vi "handle.vi"(5 "TCP connection":refnum<k5>, 7 "response queue":refnum<queue>, 10 "application request in":T1, 11 "http responder in":refnum<class "http responder.lvclass">) -> (0 "stop processing":bool, 3 "http responder out":refnum<class "http responder.lvclass">)   [LabVIEW 2013, in "http responder.lvclass"]
uses:
  http responder.lvclass
  HTTP server/http response.ctl
  HTTP server/http response packet type.ctl
  HTTP headers/http header data.ctl
  HTTP server/http request.ctl
  HTTP server/http method.ctl
  URI/url structure.ctl
  HTTP server/Basic HTTP server.lvclass
  HTTP headers/http headers.lvlib
  URI/uniform resource locator.lvlib
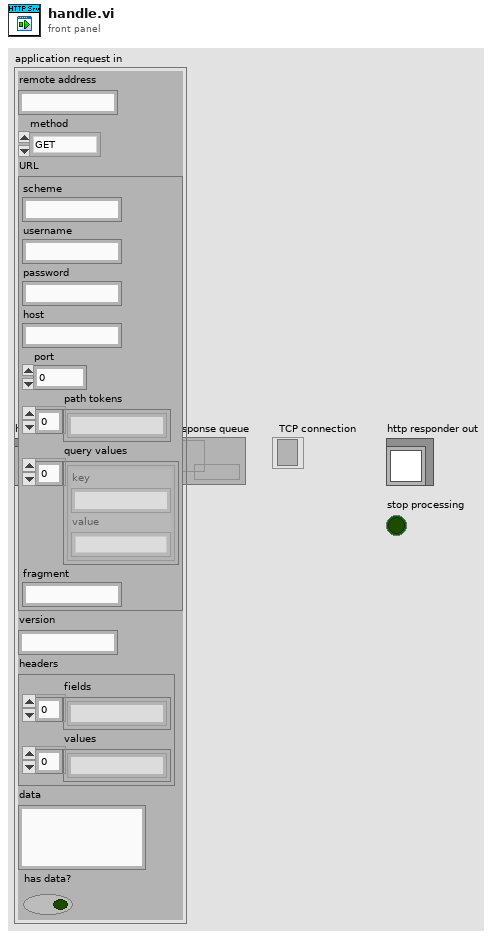
[diagram p1: front panel]
types:
  T1 = typedef "Basic HTTP server.lvclass/http request.ctl" = cluster{"remote address":string, "method":T2, "URL":T3, "version":string, "headers":T4, "data":string, "has data?":bool}
  T2 = typedef "Basic HTTP server.lvclass/http method.ctl" = enum16{"GET", "POST", "PUT", "DELETE", "HEAD", "OPTIONS", "upgrade"}
  T3 = typedef "uniform resource locator.lvlib/url structure.ctl" = cluster{"scheme":string, "username":string, "password":string, "host":string, "port":u16, "path tokens":string[], "query values":cluster{"key":string, "value":string}[], "fragment":string}
  T4 = typedef "http headers.lvlib/http header data.ctl" = cluster{"fields":string[], "values":string[]}
  T5 = typedef "Basic HTTP server.lvclass/http response packet type.ctl" = enum16{"full response", "header only", "data only", "last data"}
  T6 = typedef "Basic HTTP server.lvclass/http response.ctl" = cluster{"packet type":T5, "reason code":u16, "status string":string, "headers":T4, "cookies":string[], "data":string}
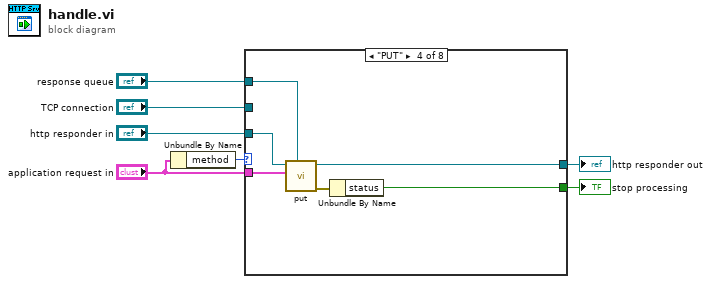
[diagram p0: block diagram]
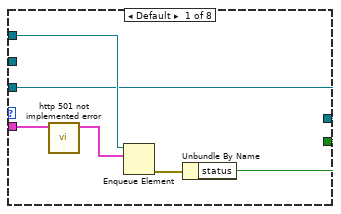
[diagram p2: hidden frame]
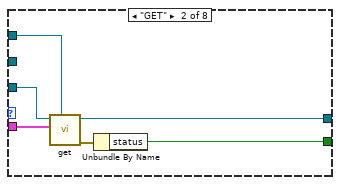
[diagram p3: hidden frame]
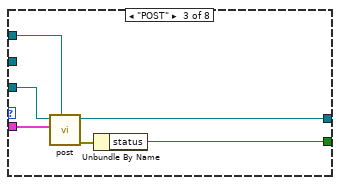
[diagram p4: hidden frame]
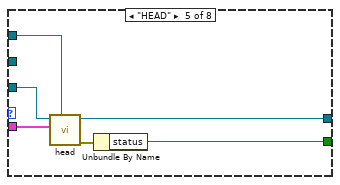
[diagram p5: hidden frame]
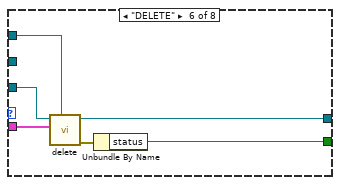
[diagram p6: hidden frame]
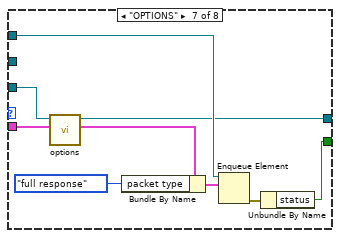
[diagram p7: hidden frame]
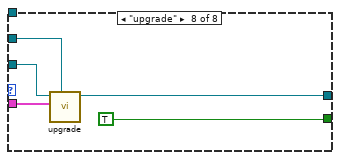
[diagram p8: hidden frame]
diagram:
  n1 = Unbundle By Name("application request in") -> ("method"=w3:T2)
  n2 = case shown="\"PUT\"" w3 {
    tunnel: "application request in" -> [w13 w14 w20 w26 w32 w38 w45 w54]
    tunnel: [w9 w19 w25 w31 w37 w43 w50 TRUE ("status")] -> w7
    tunnel: "response queue" -> [w11 w15 w21 w27 w33 w39 w51 _]
    tunnel: "TCP connection" -> [_ _ _ _ _ _ _ w53]
    tunnel: "http responder in" -> [w8 w18 w24 w30 w36 w42 w47 w56]
    tunnel: [w8 w17 w23 w29 w35 w41 w44 w55] -> w1
    frame Default {
      n3 = call "http 501 not implemented error.vi"("application request in"=w13) -> ("application request out"=w10:T6)  [unwired: 10 in]
      n4 = Enqueue Element(queue=w11, element=w10) -> (error out=w12:errorcluster)  [unwired: 2 in, 2 out]
      n5 = Unbundle By Name(w12) -> ("status"=w9:bool)
    }
    frame "GET" {
      n6 = call-dynamic "get.vi"("transmit queue"=w15, "application request in"=w14, "http responder in"=w18) -> ("error out"=w16:errorcluster, "http responder out"=w17:refnum<class "http responder.lvclass">)  [unwired: 7 in]
      n7 = Unbundle By Name(w16) -> ("status"=w19:bool)
    }
    frame "POST" {
      n8 = call-dynamic "post.vi"("transmit queue"=w21, "application request in"=w20, "http responder in"=w24) -> ("error out"=w22:errorcluster, "http responder out"=w23:refnum<class "http responder.lvclass">)  [unwired: 7 in]
      n9 = Unbundle By Name(w22) -> ("status"=w25:bool)
    }
    frame "PUT" {
      n10 = call-dynamic "put.vi"("transmit queue"=w27, "application request in"=w26, "http responder in"=w30) -> ("error out"=w28:errorcluster, "http responder out"=w29:refnum<class "http responder.lvclass">)  [unwired: 7 in]
      n11 = Unbundle By Name(w28) -> ("status"=w31:bool)
    }
    frame "HEAD" {
      n12 = call-dynamic "head.vi"("transmit queue"=w33, "application request in"=w32, "http responder in"=w36) -> ("error out"=w34:errorcluster, "http responder out"=w35:refnum<class "http responder.lvclass">)  [unwired: 7 in]
      n13 = Unbundle By Name(w34) -> ("status"=w37:bool)
    }
    frame "DELETE" {
      n14 = call-dynamic "delete.vi"("transmit queue"=w39, "application request in"=w38, "http responder in"=w42) -> ("error out"=w40:errorcluster, "http responder out"=w41:refnum<class "http responder.lvclass">)  [unwired: 7 in]
      n15 = Unbundle By Name(w40) -> ("status"=w43:bool)
    }
    frame "OPTIONS" {
      n16 = call-dynamic "options.vi"("application request in"=w45, "http responder in"=w47) -> ("application response out"=w46:T6, "http responder out"=w44:refnum<class "http responder.lvclass">)  [unwired: 8 in]
      n17 = Bundle By Name(cluster=w46, "packet type"=http_response_packet_type."full response") -> (w49:T6)
      n18 = Enqueue Element(queue=w51, element=w49) -> (error out=w52:errorcluster)  [unwired: 2 in, 2 out]
      n19 = Unbundle By Name(w52) -> ("status"=w50:bool)
    }
    frame "upgrade" {
      n20 = call "upgrade.vi"("tcp conn"=w53, "application request in"=w54, "http responder in"=w56) -> ("http responder out"=w55:refnum<class "http responder.lvclass">)  [unwired: 8 in]
    }
  }
  "http responder out" <- w1
  "stop processing" <- w7
